vi "Test_ConstructTransport_InvalidQueue_ReturnError.vi"(8 "error in (no error)":errorcluster, 11 "TestCase in":refnum<class "TestActorMessageTransport.lvclass">) -> (0 "error out":errorcluster, 3 "TestCase out":refnum<class "TestActorMessageTransport.lvclass">)   [LabVIEW 2017, in "TestActorMessageTransport.lvclass"]
uses:
  TestActorMessageTransport.lvclass
  <vilib>/ActorFramework/Message Enqueuer/Message Enqueuer.lvclass
  MockNotificationMsg/MockNotificationMsg.lvclass/MockNotificationMsg.ctl
  Source/Concrete/ActorMessageTransport/ActorMessageTransport.lvclass/ActorMessageTransport.ctl
  <vilib>/ActorFramework/Message Enqueuer/Equals Not A Refnum.vi
  MockNotificationMsg/MockNotificationMsg.lvclass
  C:/Git/composed-transport/Source/Concrete/ActorMessageTransport/Notification Msg/Notification Msg.lvclass
  <vilib>/Utility/error.llb/Error Cluster From Error Code.vi
  Source/Concrete/ActorMessageTransport/ActorMessageTransport.lvclass
  Source/Concrete/ActorMessageTransport/Notification Msg/Notification Msg.lvclass
panel:
  out "Return Error":errorcluster
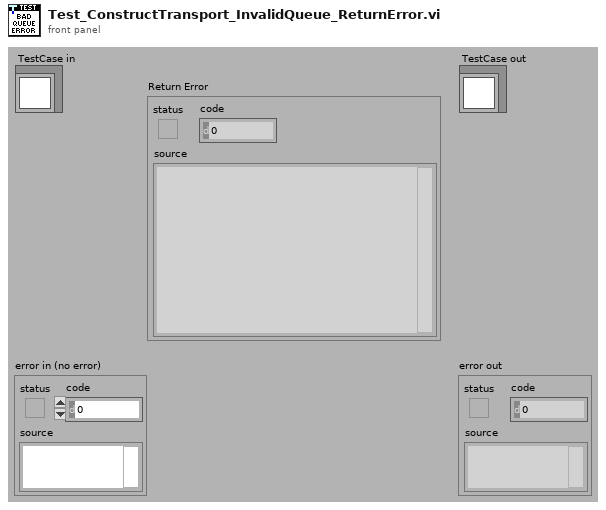
[diagram p1: front panel]
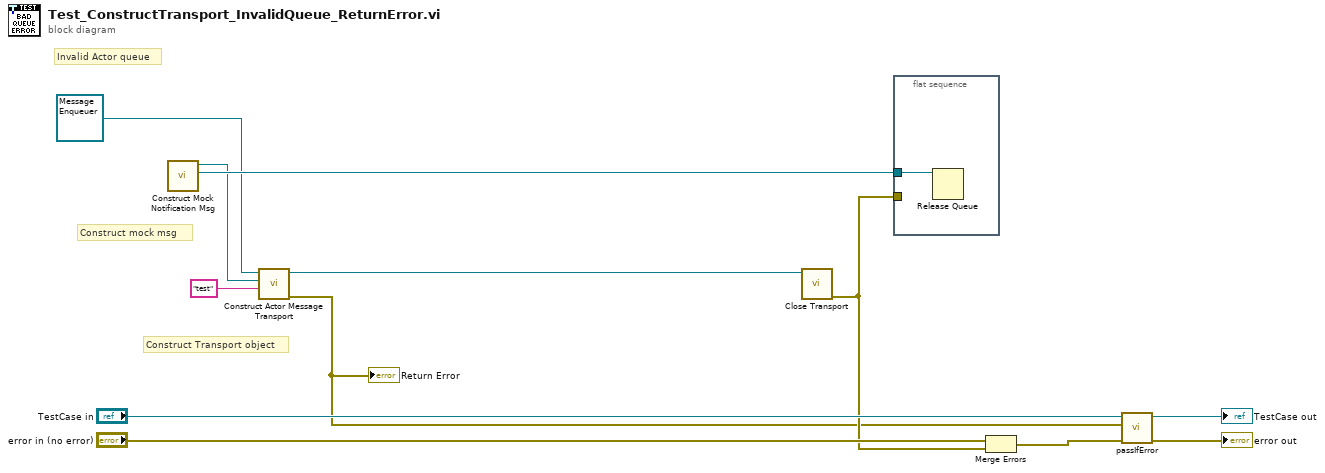
[diagram p0: block diagram]
diagram:
  # "Invalid Actor queue"
  # "Construct Transport object"
  # "Construct mock msg"
  n1 = call "Construct Mock Notification Msg.vi"() -> ("Data leak test queue"=w6:refnum<queue>, "MockNotificationMsg out"=w4:refnum<class "MockNotificationMsg.lvclass">)  [unwired: 9 in, 1 out]
  n2 = call "Construct Actor Message Transport.vi"("Datum Name"="test", "Notification Msg"=w4, "Message Enqueuer in"=refnum<class "Message Enqueuer.lvclass"> refnum ("Self Enqueuer")) -> ("error out"=w1:errorcluster, "ActorMessageTransport"=w2:refnum<class "ActorMessageTransport.lvclass">)  [unwired: 7 in]
  "Return Error" <- w1
  n3 = call-dynamic "Close Transport.vi"("ITransport in"=w2) -> ("error out"=w5:errorcluster)  [unwired: 10 in]
  n4 = flat-sequence {
    tunnel: w6 -> [w13]
    tunnel: w5 -> [_]
    frame #0 {
      n5 = Release Queue(queue=w13) -> ()  [unwired: 2 in, 3 out]
    }
  }
  n6 = Merge Errors("error in (no error)", w5) -> (w8:errorcluster)
  n7 = call-dynamic "passIfError.vi"("error in (no error)"=w8, "error"=w1, "TestCase in"="TestCase in") -> ("error out"=→"error out":errorcluster, "TestCase out"=→"TestCase out":refnum<class "TestActorMessageTransport.lvclass">)  [unwired: 7 in]
